vi "Choreo_Choreo_GetTrajectory.vi"(11 "FileName":string="C:\\Users\\Jim\\Desktop\\PathPlanner24\\Choreo\\ChoreoTest.TRAJ") -> (0 "error out":errorcluster, 3 "ChoreoTrajectory":T1, 4 "Full Filename":string)   [LabVIEW 2019]
doc: "Load a Choreo trajectory from a JSON formatted file. Note that for newer versions of Choreo, the file has a \".traj\" extension. Internally this is formatted as a JSON file.\n\nInputs: \n - filename - string - The name of the trajectory file. See notes below on file naming.\n\nOutputs:\n - Trajectory - cluster - Trajectory read from JSON file.\n - Error out - cluster - Error cluster\n - Full Filename - string - fully qualified file name.\n\nNotes on file naming:\n - The file name must include the extention. \".json\", or \".traj\" is not automatically appended to the name. \n - The file name can be a simple file or an absolute path. If a simple file name is used the default path on the RoboRIO is: \"home:\\lvuser\\natinst\\LabVIEW Data\". On a Windows PC the default path is the LabVIEW default directory. Normally this is: “%HOMEDRIVE%%HOMEPATH%\\Documents\\LabView Data\".\n - Filenames on the RoboRIO, which runs Linux, are case sensitive."
uses:
  TypeDef/ChoreoTrajectory.ctl
  TypeDef/ChoreoTrajectoryState.ctl
  ChoreoLib.lvlib
panel:
  in  "error in (no error)":errorcluster
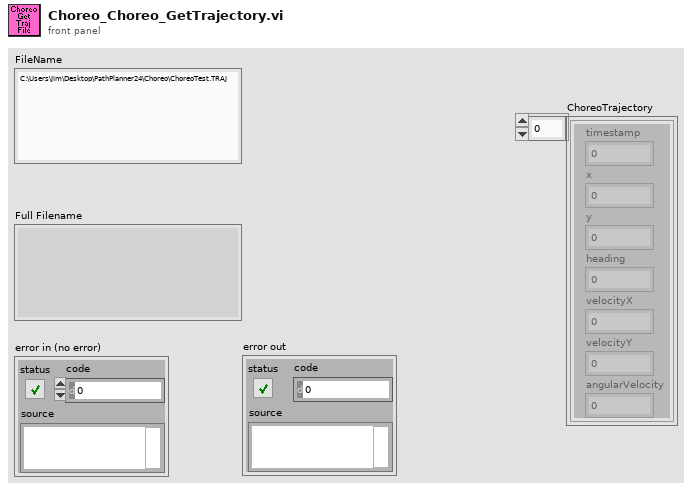
[diagram p1: front panel]
types:
  T1 = typedef "ChoreoLib.lvlib/ChoreoTrajectory.ctl" = T2[]
  T2 = typedef "ChoreoLib.lvlib/ChoreoTrajectoryState.ctl" = cluster{"timestamp":dbl, "x":dbl, "y":dbl, "heading":dbl, "velocityX":dbl, "velocityY":dbl, "angularVelocity":dbl}
  T3 = enum16{"open", "replace", "create", "open or create", "replace or create", "replace or create with confirmation"}
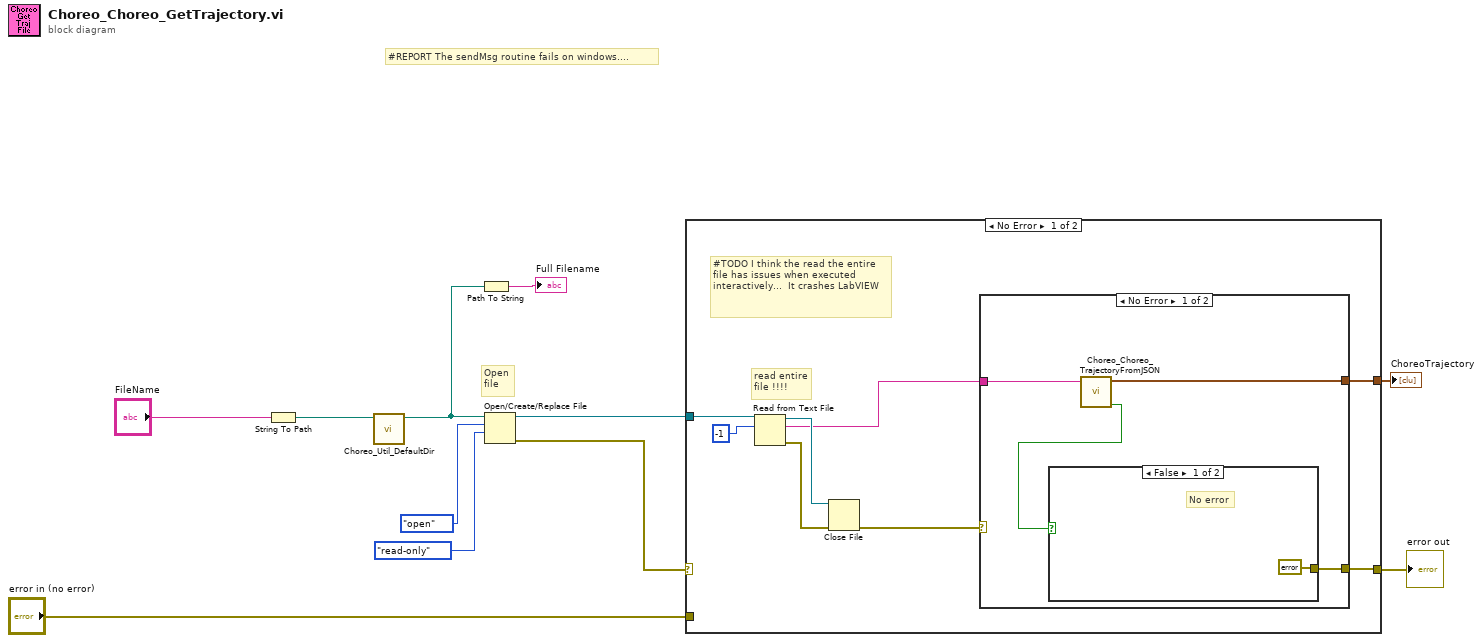
[diagram p0: block diagram]
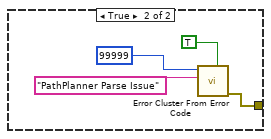
[diagram p2: hidden frame]
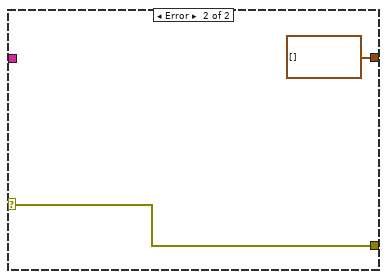
[diagram p3: hidden frame]
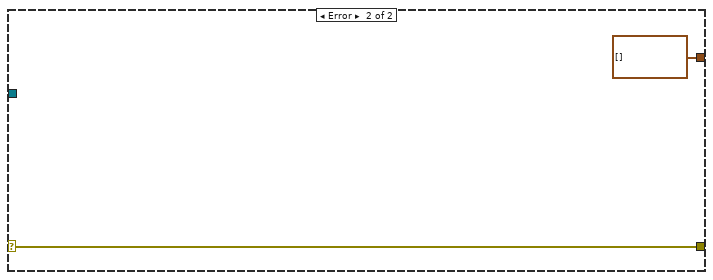
[diagram p4: hidden frame]
diagram:
  # "#REPORT The sendMsg routine fails on windows...."
  # "Open\nfile"
  n1 = String To Path(string="FileName") -> (path=w2:path)
  n2 = call "Choreo_Util_DefaultDir.vi"("Path in"=w2) -> ("Path Out"=w1:path)  [unwired: 10 in]
  n3 = Path To String(path=w1) -> (string=→"Full Filename":string)
  n4 = Open/Create/Replace File(file path (use dialog)=w1, operation (0:open)=T3."open", access (0:read/write)=enum16{"read/write", "read-only", "write-only"}."read-only") -> (refnum out=w7:refnum<file>, error out=w9:errorcluster)  [unwired: 3 in, 1 out]
  n5 = case shown="No Error" w9 {
    selector: w9 -> [_ w32]
    tunnel: w7 -> [w18 _]
    tunnel: [w13 w32] -> w4
    tunnel: "error in (no error)" -> [_ _]
    tunnel: [w12 T1 [] ("ChoreoTrajectory")] -> w3
    frame No Error {
      # "#TODO I think the read the entire\nfile has issues when executed\ninteractively...  It crashes LabVIEW"
      # "read entire\nfile !!!!"
      n6 = Read from Text File(file (use dialog)=w18, count=-1) -> (refnum out=w17:refnum<file>, text=w16:string, error out=w15:errorcluster)  [unwired: 2 in, 1 out]
      n7 = Close File(refnum=w17, error in=w15) -> (error out=w14:errorcluster)  [unwired: 1 out]
      n8 = case shown="No Error" w14 {
        selector: w14 -> [_ w30]
        tunnel: w16 -> [w23 _]
        tunnel: [w21 w30] -> w13
        tunnel: [w20 T1 [] ("ChoreoTrajectory")] -> w12
        frame No Error {
          n9 = call "Choreo_Choreo_TrajectoryFromJSON.vi"("JSON String"=w23) -> ("Error"=w22:bool, "ChoreoTrajectory"=w20:T1)  [unwired: 9 in]
          n10 = case shown="False" w22 {
            tunnel: [errorcluster {"status"=FALSE, "code"=0, "source"=""} ("error out") w25] -> w21
            frame False {
              # "No error"
            }
            frame True {
              n11 = call <vilib>:"Error Cluster From Error Code.vi"("is warning? (False)"=TRUE, "error message (\"\")"="PathPlanner Parse Issue" ("error message (\"\")"), "error code (0)"=99999) -> ("error out"=w25:errorcluster)  [unwired: 6 in]
            }
          }
        }
        frame Error {
        }
      }
    }
    frame Error {
    }
  }
  "error out" <- w4
  "ChoreoTrajectory" <- w3
